vi "decimater.vi"() -> ()   [LabVIEW 2020]
uses:
  classes/hardware-protocol/serial/HP-S-data.ctl
  classes/hardware-protocol/serial/HP-S-Serial.lvclass
panel:
  out "reversed array":T1 format="%x"
  out "Numeric 2":i32
  out "x-y":u32
  out "first subarray 5":T2(array[cluster])
  out "size(s) 10":i32
  out "size(s) 9":i32
  out "first subarray 4":T2(array[cluster])
  out "size(s) 8":i32
  out "size(s) 7":i32
  out "first subarray 3":T2(array[cluster])
  out "size(s) 6":i32
  out "Numeric":i32
  out "second subarray":T2(array[cluster])
  out "Waveform Graph 3":dbl[][](graph)
  out "length 3":i32
  out "floor(x/y)":i32
  out "x-y*floor(x/y)":i32
  out "size(s) 5":i32
  out "Waveform Graph 2":dbl[][](graph)
  out "value 2":T2(array[cluster])
  out "size(s) 4":i32
  out "Array 2":u16[](array[numeric])
  out "*(type *) &x":i32
  out "Waveform Graph":dbl[][](graph)
  out "decimated array 3":i32[](array[numeric])
  out "Array":i32[](array[numeric])
  out "decimated array":i32[](array[numeric])
  out "x*y":i32
  out "size(s) 2":i32
  out "size(s)":i32
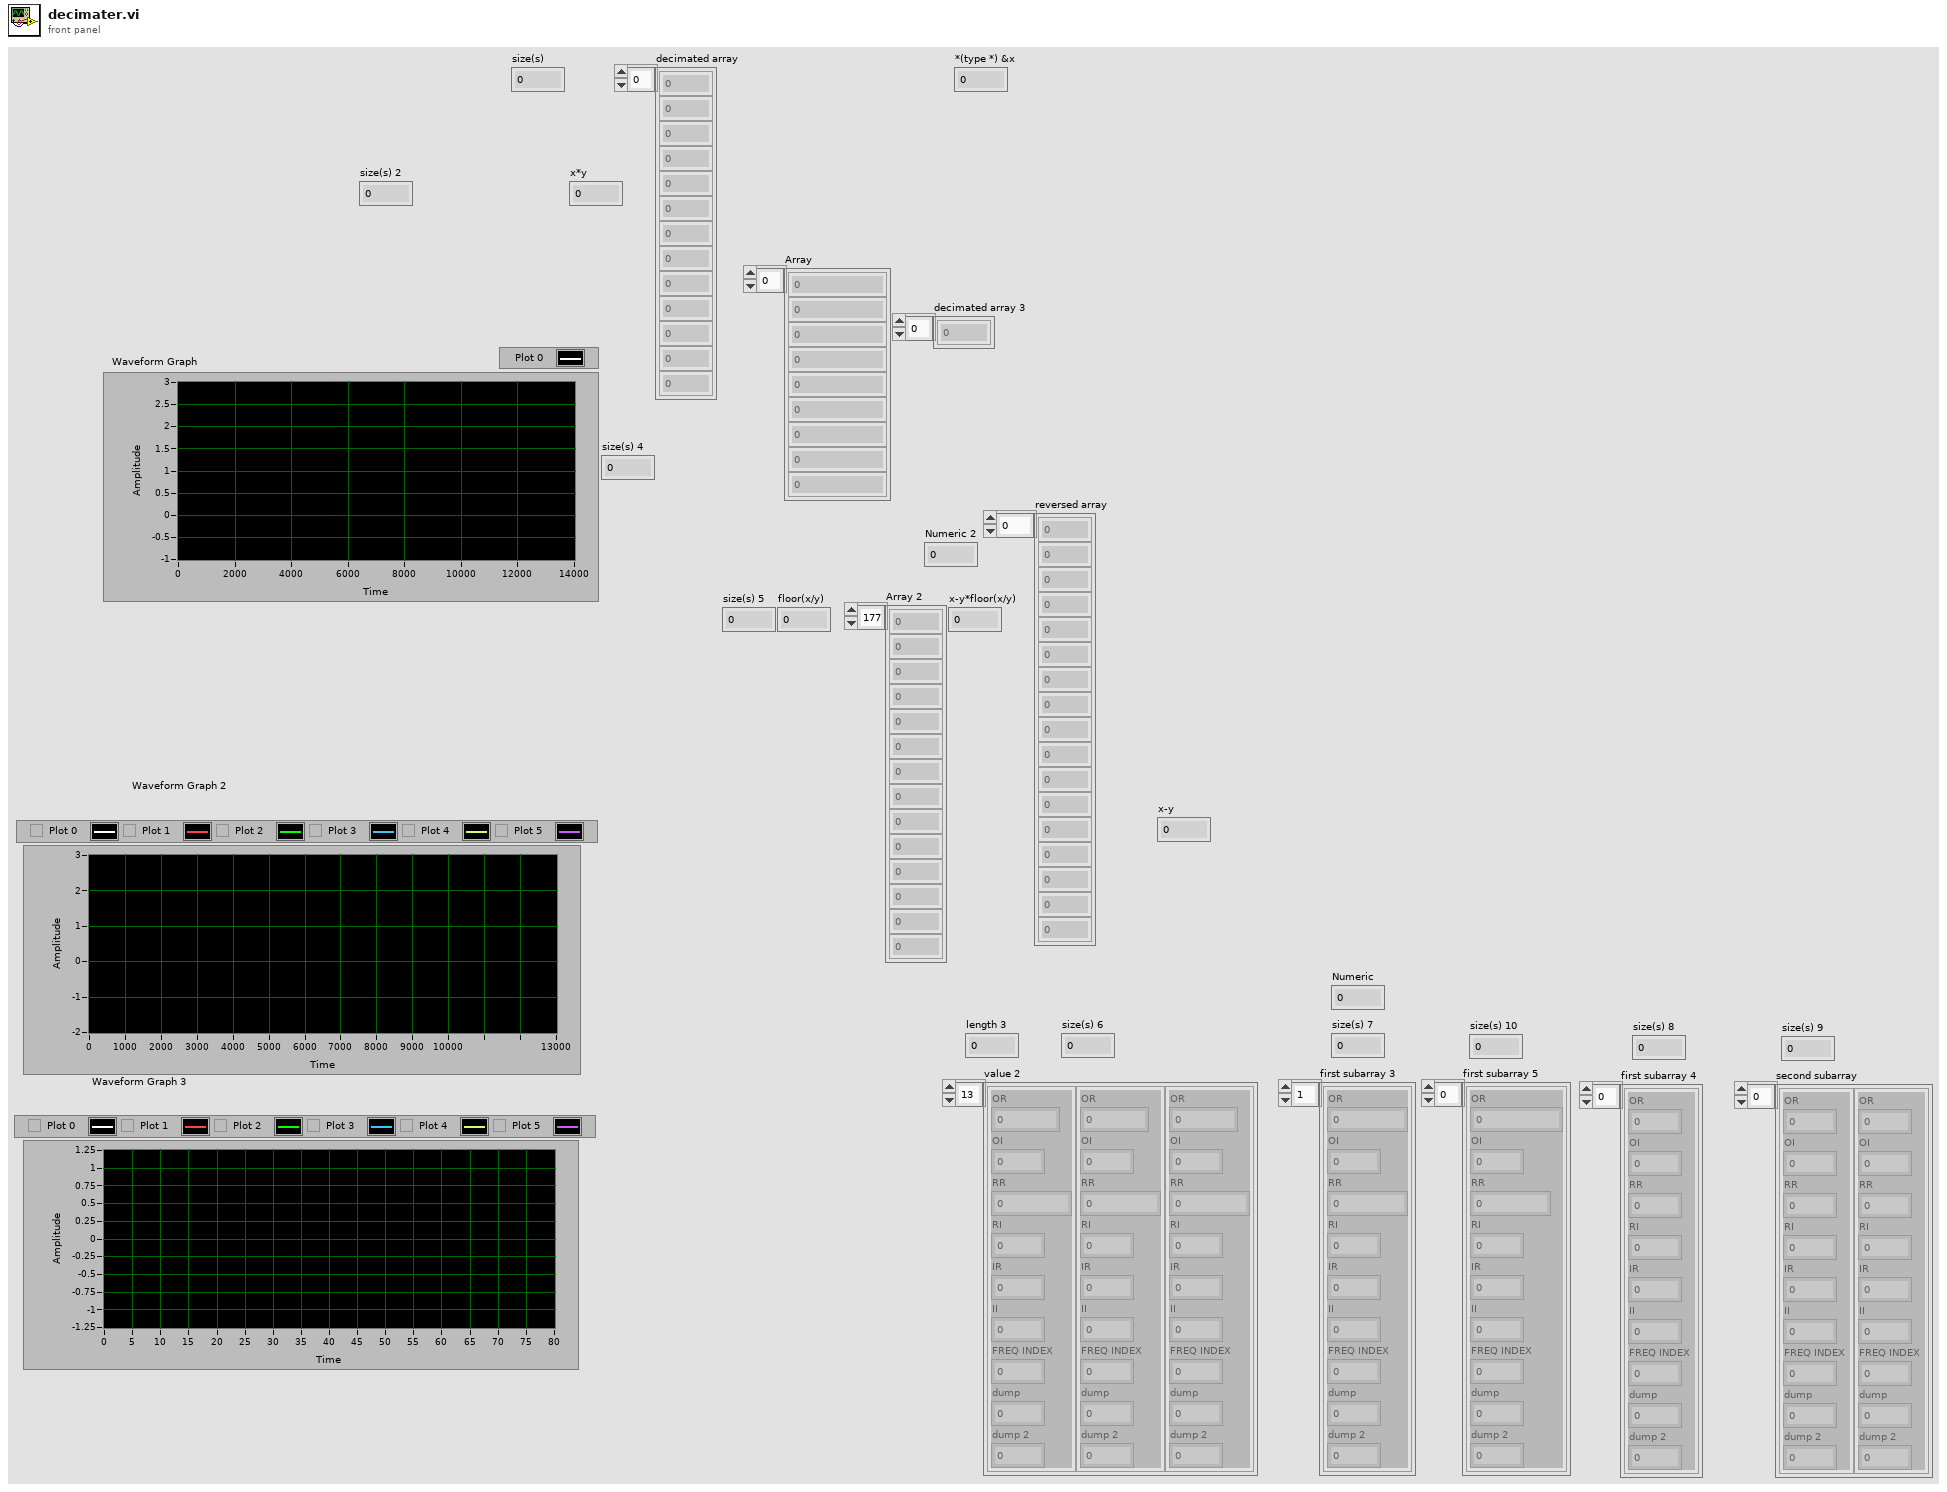
[diagram p1: front panel]
types:
  T1 = typedef "HP-S-Serial.lvclass/HP-S-data.ctl" = u8[]
  T2 = cluster{"OR":i32, "OI":i32, "RR":i32, "RI":i32, "IR":i32, "II":i32, "FREQ INDEX":u16, "dump":u16, "dump 2":u32}[]
  T3 = cluster{"OR":i32, "OI":i32, "RR":i32, "RI":i32, "IR":i32, "II":i32, "FREQ INDEX":u16, "dump":u16, "dump 2":u32}
  T4 = enum16{"big-endian, network order", "native, host order", "little-endian"}
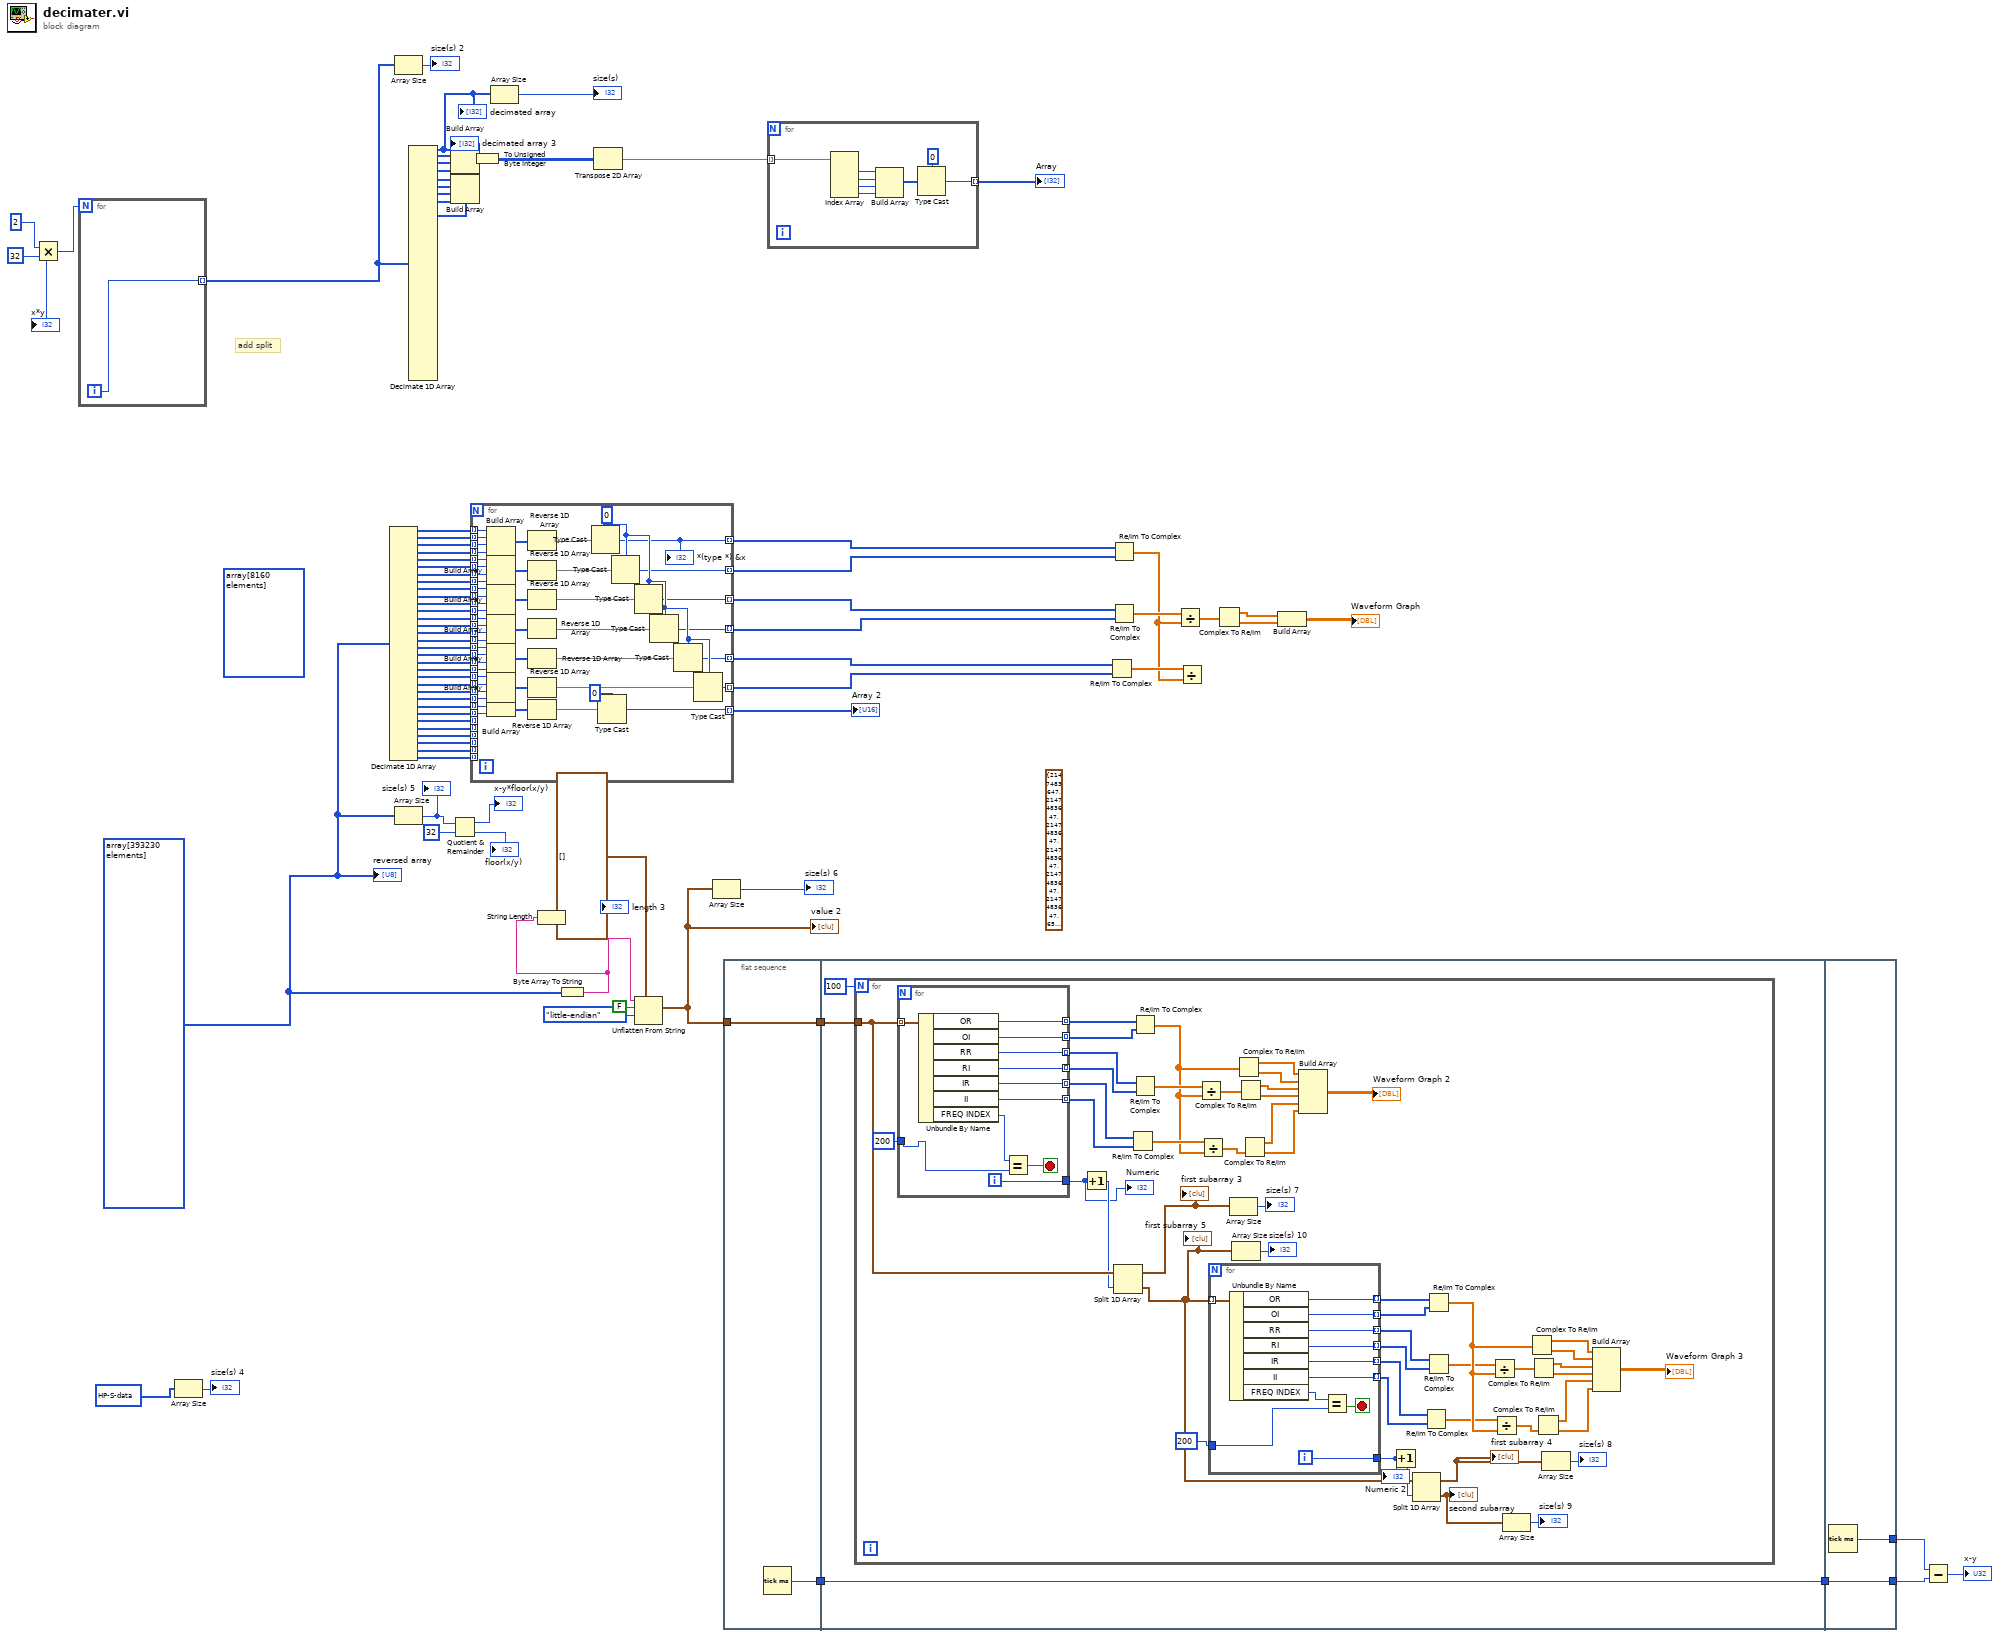
[diagram p0: block diagram]
diagram:
  w1 = T1 array[393230 elements] ("Emtpied buffer")
  (unwired) T3 {"OR"=2147483647, "OI"=2147483647, "RR"=2147483647, "RI"=2147483647, "IR"=2147483647, "II"=2147483647, "FREQ INDEX"=65535, "dump"=65535, "dump 2"=2147483647} ("Cluster")
  (unwired) u8[] array[8160 elements] ("unsigned byte array 3")
  # "add split"
  n1 = Multiply(x=2, y=32) -> (x*y=w83:i32)
  "x*y" <- w83
  n2 = for {
    N: w83 -> [_]
    tunnel: [w86] -> w80 mode=indexing
    i -> [w86]
  }
  n3 = Array Size(array=T1 [0, 0, 0, 64, 0, 0, 0, 0, 128, 9, 212, 201, 192, 252, 118, 3, 35, 211, 255, 255, 129, 41, 0, 0, 77, 0, 0, 0, 0, 0, 0, 161, 0, 0, 0, 64, 0, 0, 0, 0, 128, 42, 38, 202, 72, 130, 232, 6, 70, 37, 0, 0, 166, 175, 0, 0, 78, 0, 0, 0, 0, 0, 0, 127, 0, 0, 0, 64, 0, 0, 0, 0, 128, 192, 193, 202, 16, 252, 87, 10] ("read buffer")) -> (size(s)=→"size(s) 4":i32)
  n4 = Decimate 1D Array(w1) -> (w66:T1, w65:T1, w64:T1, w63:T1, w62:T1, w61:T1, w60:T1, w59:T1, w58:T1, w57:T1, w56:T1, w55:T1, w54:T1, w53:T1, w52:T1, w51:T1, w50:T1, w49:T1, w48:T1, w47:T1, w46:T1, w45:T1, w44:T1, w43:T1, w42:T1, w41:T1, w40:T1, w39:T1, w38:T1, w37:T1, w36:T1, w35:T1)
  n5 = Array Size(array=w80) -> (size(s)=→"size(s) 2":i32)
  n6 = Array Size(array=w1) -> (size(s)=w15:i32)
  "size(s) 5" <- w15
  n7 = Decimate 1D Array(w80) -> (w79:i32[], w78:i32[], w77:i32[], w76:i32[], w75:i32[], w74:i32[], w73:i32[], w72:i32[], →"decimated array 3":i32[])  [unwired: 23 out]
  "decimated array" <- w79
  n8 = Build Array(w79, w78, w77, w76) -> (w71:i32[][])
  n9 = Build Array(w75, w74, w73, w72) -> ()  [unwired: 1 out]
  n10 = Quotient & Remainder(x=w15, y=32) -> (x-y*floor(x/y)=→"x-y*floor(x/y)":i32, floor(x/y)=→"floor(x/y)":i32)
  n11 = for {
    tunnel: w66 -> [w135] mode=indexing
    tunnel: w65 -> [w134] mode=indexing
    tunnel: w64 -> [w133] mode=indexing
    tunnel: w63 -> [w132] mode=indexing
    tunnel: w62 -> [w131] mode=indexing
    tunnel: w61 -> [w130] mode=indexing
    tunnel: w60 -> [w129] mode=indexing
    tunnel: w59 -> [w128] mode=indexing
    tunnel: w58 -> [w127] mode=indexing
    tunnel: w57 -> [w126] mode=indexing
    tunnel: w56 -> [w125] mode=indexing
    tunnel: w55 -> [w124] mode=indexing
    tunnel: w54 -> [w123] mode=indexing
    tunnel: w53 -> [w122] mode=indexing
    tunnel: w52 -> [w121] mode=indexing
    tunnel: w51 -> [w120] mode=indexing
    tunnel: w50 -> [w119] mode=indexing
    tunnel: w49 -> [w118] mode=indexing
    tunnel: w48 -> [w117] mode=indexing
    tunnel: w47 -> [w116] mode=indexing
    tunnel: w46 -> [w115] mode=indexing
    tunnel: w45 -> [w114] mode=indexing
    tunnel: w44 -> [w113] mode=indexing
    tunnel: w43 -> [w112] mode=indexing
    tunnel: w42 -> [w98] mode=indexing
    tunnel: w41 -> [w97] mode=indexing
    tunnel: w40 -> [_] mode=indexing
    tunnel: w39 -> [_] mode=indexing
    tunnel: w38 -> [_] mode=indexing
    tunnel: w37 -> [_] mode=indexing
    tunnel: w36 -> [_] mode=indexing
    tunnel: w35 -> [_] mode=indexing
    tunnel: [w104] -> w34 mode=indexing
    tunnel: [w103] -> w33 mode=indexing
    tunnel: [w102] -> w32 mode=indexing
    tunnel: [w101] -> w31 mode=indexing
    tunnel: [w100] -> w30 mode=indexing
    tunnel: [w99] -> w29 mode=indexing
    tunnel: [w94] -> w21 mode=indexing
    w105 = 0
    n12 = Build Array(w135, w134, w133, w132) -> (w110:u8[])
    n13 = Build Array(w131, w130, w129, w128) -> (w111:u8[])
    n14 = Build Array(w127, w126, w125, w124) -> (w109:u8[])
    n15 = Build Array(w123, w122, w121, w120) -> (w108:u8[])
    n16 = Build Array(w119, w118, w117, w116) -> (w107:u8[])
    n17 = Build Array(w115, w114, w113, w112) -> (w106:u8[])
    n18 = Build Array(w98, w97) -> (w96:u8[])
    n19 = Reverse 1D Array(array=w110) -> (reversed array=w93:u8[])
    n20 = Reverse 1D Array(array=w111) -> (reversed array=w92:u8[])
    n21 = Reverse 1D Array(array=w109) -> (reversed array=w91:u8[])
    n22 = Reverse 1D Array(array=w108) -> (reversed array=w90:u8[])
    n23 = Reverse 1D Array(array=w107) -> (reversed array=w89:u8[])
    n24 = Reverse 1D Array(array=w106) -> (reversed array=w88:u8[])
    n25 = Reverse 1D Array(array=w96) -> (reversed array=w87:u8[])
    n26 = Type Cast(type=w105, x=w93) -> (*(type *) &x=w104:i32)
    "*(type *) &x" <- w104
    n27 = Type Cast(type=u16 0, x=w87) -> (*(type *) &x=w94:u16)
    n28 = Type Cast(type=w105, x=w92) -> (*(type *) &x=w103:i32)
    n29 = Type Cast(type=w105, x=w91) -> (*(type *) &x=w102:i32)
    n30 = Type Cast(type=w105, x=w90) -> (*(type *) &x=w101:i32)
    n31 = Type Cast(type=w105, x=w89) -> (*(type *) &x=w100:i32)
    n32 = Type Cast(type=w105, x=w88) -> (*(type *) &x=w99:i32)
  }
  "Array 2" <- w21
  n33 = To Unsigned Byte Integer(number=w71) -> (unsigned 8bit integer=w68:u8[][])
  n34 = Array Size(array=w79) -> (size(s)=→"size(s)":i32)
  n35 = Byte Array To String(unsigned byte array=w1) -> (string=w11:string)
  n36 = String Length(string=w11) -> (length=→"length 3":i32)
  n37 = Transpose 2D Array(2D array=w68) -> (transposed array=w69:u8[][])
  n38 = Unflatten From String(type=T2 [], binary string=w11, data includes array or string size? (T)=FALSE, byte order (0:big-endian, network order)=T4."little-endian") -> (value=w9:T2)  [unwired: 1 in, 2 out]
  "value 2" <- w9
  n39 = Array Size(array=w9) -> (size(s)=→"size(s) 6":i32)
  n40 = flat-sequence {
    tunnel: w9 -> [w137]
    tunnel: [w137] -> w7
    tunnel: [w136] -> w5
    tunnel: w7 -> [w140]
    tunnel: [w139] -> w6
    tunnel: w5 -> [w139]
    tunnel: [w215] -> w4
    tunnel: w6 -> [w215]
    tunnel: [w214] -> w3
    frame #0 {
      n41 = Tick Count (ms)() -> (millisecond timer value=w136:u32)
    }
    frame #1 {
      n42 = for {
        N: 100 -> [_]
        tunnel: w140 -> [w154]
        n43 = for {
          tunnel: w154 -> [w213] mode=indexing
          tunnel: [w212] -> w186 mode=indexing
          tunnel: [w211] -> w185 mode=indexing
          tunnel: [w210] -> w184 mode=indexing
          tunnel: [w209] -> w183 mode=indexing
          tunnel: [w208] -> w182 mode=indexing
          tunnel: [w207] -> w181 mode=indexing
          tunnel: [w205] -> w141
          tunnel: u16 200 ("FREQ INDEX") -> [w203]
          i -> [w205]
          stop <- w204 stop-if-true
          n44 = Unbundle By Name(w213) -> ("OR"=w212:i32, "OI"=w211:i32, "RR"=w210:i32, "RI"=w209:i32, "IR"=w208:i32, "II"=w207:i32, "FREQ INDEX"=w206:u16)
          n45 = Equal?(x=w206, y=w203) -> (x = y?=w204:bool)
        }
        "Numeric" <- w141
        n46 = Increment(x=w141) -> (x+1=w143:i32)
        n47 = Split 1D Array(array=w154, index=w143) -> (first subarray=w151:T2, second subarray=w144:T2)
        "first subarray 3" <- w151
        "first subarray 5" <- w144
        n48 = Re/Im To Complex(1:w181, 2:w182) -> (0:w188:cdb[])
        n49 = Re/Im To Complex(1:w185, 2:w186) -> (0:w176:cdb[])
        n50 = Re/Im To Complex(1:w183, 2:w184) -> (0:w187:cdb[])
        n51 = Divide(x=w187, y=w176) -> (x/y=w177:cdb[])
        n52 = Divide(x=w188, y=w176) -> (x/y=w180:cdb[])
        n53 = for {
          tunnel: w144 -> [w202] mode=indexing
          tunnel: [w201] -> w161 mode=indexing
          tunnel: [w200] -> w162 mode=indexing
          tunnel: [w199] -> w163 mode=indexing
          tunnel: [w198] -> w164 mode=indexing
          tunnel: [w197] -> w165 mode=indexing
          tunnel: [w196] -> w166 mode=indexing
          tunnel: [w194] -> w155
          tunnel: u16 200 ("FREQ INDEX") -> [w192]
          i -> [w194]
          stop <- w193 stop-if-true
          n54 = Unbundle By Name(w202) -> ("OR"=w201:i32, "OI"=w200:i32, "RR"=w199:i32, "RI"=w198:i32, "IR"=w197:i32, "II"=w196:i32, "FREQ INDEX"=w195:u16)
          n55 = Equal?(x=w195, y=w192) -> (x = y?=w193:bool)
        }
        "Numeric 2" <- w155
        n56 = Array Size(array=w151) -> (size(s)=→"size(s) 7":i32)
        n57 = Array Size(array=w144) -> (size(s)=→"size(s) 10":i32)
        n58 = Complex To Re/Im(x + iy=w176) -> (x=w174:dbl[], y=w175:dbl[])
        n59 = Complex To Re/Im(x + iy=w177) -> (x=w189:dbl[], y=w190:dbl[])
        n60 = Complex To Re/Im(x + iy=w180) -> (x=w179:dbl[], y=w178:dbl[])
        n61 = Build Array(w174, w175, w189, w190, w179, w178) -> (→"Waveform Graph 2":dbl[][])
        n62 = Increment(x=w155) -> (x+1=w142:i32)
        n63 = Split 1D Array(array=w144, index=w142) -> (first subarray=w148:T2, second subarray=w146:T2)
        "second subarray" <- w146
        "first subarray 4" <- w148
        n64 = Re/Im To Complex(1:w166, 2:w165) -> (0:w159:cdb[])
        n65 = Re/Im To Complex(1:w162, 2:w161) -> (0:w171:cdb[])
        n66 = Re/Im To Complex(1:w164, 2:w163) -> (0:w160:cdb[])
        n67 = Divide(x=w160, y=w171) -> (x/y=w170:cdb[])
        n68 = Divide(x=w159, y=w171) -> (x/y=w167:cdb[])
        n69 = Array Size(array=w146) -> (size(s)=→"size(s) 9":i32)
        n70 = Complex To Re/Im(x + iy=w171) -> (x=w173:dbl[], y=w172:dbl[])
        n71 = Complex To Re/Im(x + iy=w170) -> (x=w158:dbl[], y=w157:dbl[])
        n72 = Complex To Re/Im(x + iy=w167) -> (x=w168:dbl[], y=w169:dbl[])
        n73 = Array Size(array=w148) -> (size(s)=→"size(s) 8":i32)
        n74 = Build Array(w173, w172, w158, w157, w168, w169) -> (→"Waveform Graph 3":dbl[][])
      }
    }
    frame #2 {
      n75 = Tick Count (ms)() -> (millisecond timer value=w214:u32)
    }
  }
  n76 = for {
    tunnel: w69 -> [w223] mode=indexing
    tunnel: [w216] -> w70 mode=indexing
    n77 = Index Array(array=w223) -> (element #1=w222:u8, element #2=w221:u8, element #3=w220:u8, element #4=w219:u8)  [unwired: 4 in]
    n78 = Build Array(w222, w221, w220, w219) -> (w218:u8[])
    n79 = Type Cast(type=0, x=w218) -> (*(type *) &x=w216:i32)
  }
  "Array" <- w70
  n80 = Re/Im To Complex(1:w29, 2:w30) -> (0:w27:cdb[])
  n81 = Re/Im To Complex(1:w33, 2:w34) -> (0:w26:cdb[])
  n82 = Re/Im To Complex(1:w31, 2:w32) -> (0:w28:cdb[])
  n83 = Divide(x=w28, y=w26) -> (x/y=w25:cdb[])
  n84 = Divide(x=w27, y=w26) -> ()  [unwired: 1 out]
  n85 = Complex To Re/Im(x + iy=w25) -> (x=w24:dbl[], y=w23:dbl[])
  n86 = Build Array(w24, w23) -> (→"Waveform Graph":dbl[][])
  n87 = Subtract(x=w3, y=w4) -> (x-y=→"x-y":u32)
  "reversed array" <- w1
